vi "Read Results.vi"(8 "error in (no error)":errorcluster, 11 "Results List in":refnum<class "Results List.lvclass">) -> (0 "error out":errorcluster, 2 "Results":refnum<class "Result.lvclass">[](array[class]), 3 "Results List out":refnum<class "Results List.lvclass">)   [LabVIEW 2015, in "Results List.lvclass"]
uses:
  Results List.lvclass
  Result/Result.lvclass
  Results List.lvclass/Results List.ctl
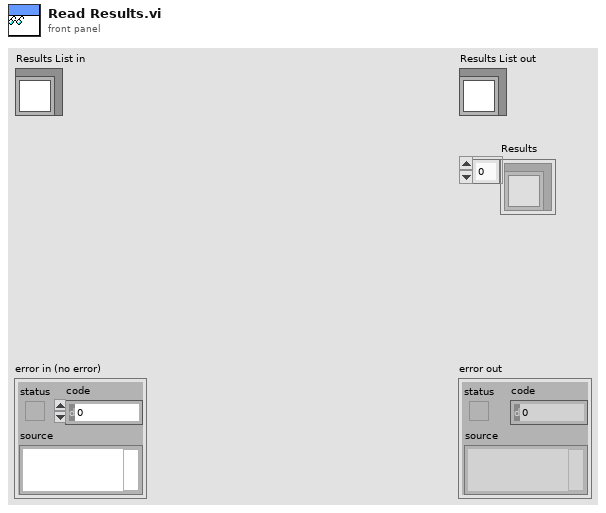
[diagram p1: front panel]
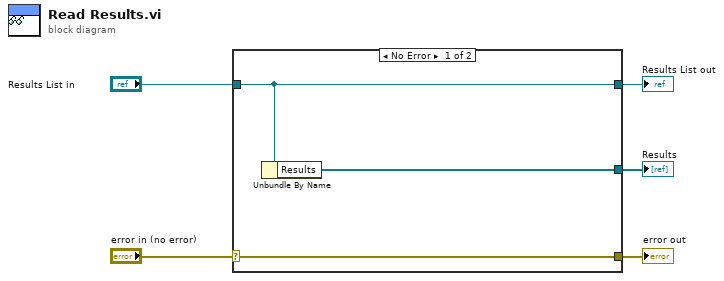
[diagram p0: block diagram]
diagram:
  n1 = case shown="No Error" "error in (no error)" {
    selector: "error in (no error)" -> [w8 w9]
    tunnel: [w8 w9] -> w4
    tunnel: [w7 w10] -> w2
    tunnel: "Results List in" -> [w7 w10]
    tunnel: [w6 _] -> w1
    frame No Error {
      n2 = Unbundle By Name(w7) -> ("Results"=w6:refnum<class "Result.lvclass">[])
    }
    frame Error {
    }
  }
  "error out" <- w4
  "Results List out" <- w2
  "Results" <- w1
